vi "iKNearestNeighbors.vi"(4 "Nominal End":i32, 6 "Nominal Start":i32, 8 "Index":i32, 9 "Span":i32, 10 "Weights":dbl[](array[numeric]), 11 "X":dbl[](array[numeric])) -> (3 "Nearest Neighbors Mask":bool[](array[boolean]))   [LabVIEW 2020]
uses:
  Array Manipulation VIs/Irregular Array Subset (DBL).vi
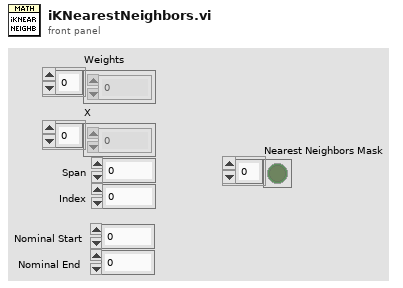
[diagram p1: front panel]
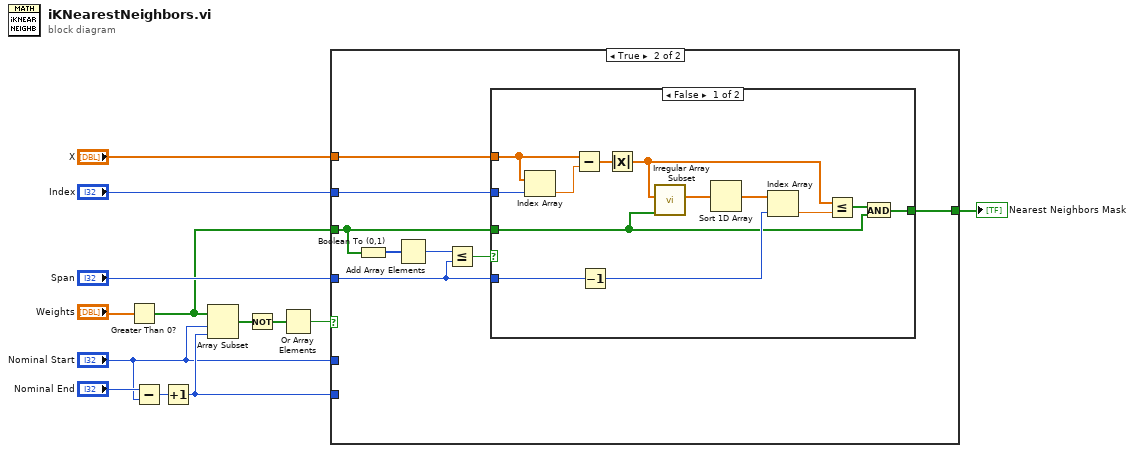
[diagram p0: block diagram]
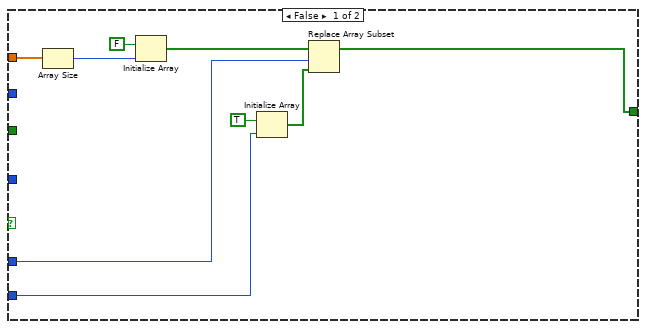
[diagram p2: hidden frame]
diagram:
  n1 = Greater Than 0?(x="Weights") -> (x > 0?=w3:bool[])
  n2 = Subtract(x="Nominal End", y="Nominal Start") -> (x-y=w9:i32)
  n3 = Increment(x=w9) -> (x+1=w2:i32)
  n4 = Array Subset(array=w3, index="Nominal Start", length=w2) -> (w6:bool[])
  n5 = Not(x=w6) -> (.not. x?=w5:bool[])
  n6 = Or Array Elements(Boolean array=w5) -> (logical OR=w4:bool)
  n7 = case shown="True" w4 {
    tunnel: "X" -> [w20 w27]
    tunnel: "Index" -> [_ w26]
    tunnel: w3 -> [_ w25]
    tunnel: "Span" -> [_ w24]
    tunnel: [w14 w23] -> w10
    tunnel: w2 -> [w18 _]
    tunnel: "Nominal Start" -> [w15 _]
    frame False {
      n8 = Array Size(array=w20) -> (size(s)=w21:i32)
      n9 = Initialize Array(FALSE, w21) -> (w17:bool[])
      n10 = Initialize Array(TRUE, w18) -> (w16:bool[])
      n11 = Replace Array Subset(array=w17, new element=w16, index=w15) -> (w14:bool[])
    }
    frame True {
      n12 = Boolean To (0,1)(Boolean=w25) -> (0, 1=w30:i16[])
      n13 = Add Array Elements(numeric array=w30) -> (sum=w29:i16)
      n14 = Less Or Equal?(x=w29, y=w24) -> (x <= y?=w28:bool)
      n15 = case shown="False" w28 {
        tunnel: w27 -> [w43 _]
        tunnel: w26 -> [w42 _]
        tunnel: w25 -> [w35 w44]
        tunnel: w24 -> [w38 _]
        tunnel: [w33 w44] -> w23
        frame False {
          n16 = Index Array(array=w43, index=w42) -> (element=w41:dbl)
          n17 = Subtract(x=w43, y=w41) -> (x-y=w40:dbl[])
          n18 = Decrement(x=w38) -> (x-1=w37:i32)
          n19 = Absolute Value(x=w40) -> (abs(x)=w31:dbl[])
          n20 = call-poly "Irregular Array Subset.vi"("Mask"=w35, "Array"=w31) -> ("Array Subset"=w34:dbl[])  [unwired: 8 in, 1 out]
          n21 = Sort 1D Array(array=w34) -> (sorted array=w39:dbl[])
          n22 = Index Array(array=w39, index=w37) -> (element=w36:dbl)
          n23 = Less Or Equal?(x=w31, y=w36) -> (x <= y?=w32:bool[])
          n24 = And(x=w32, y=w35) -> (x .and. y?=w33:bool[])
        }
        frame True {
        }
      }
    }
  }
  "Nearest Neighbors Mask" <- w10
